vi "LP RT Stream reader State Decide.vi"(8 "error in (no error)":errorcluster, 10 "RefreshRate":i32, 11 "Queue in":refnum<queue>) -> (0 "error out":errorcluster, 1 "Data":variant, 2 "CMD":T1, 3 "queue out":refnum<queue>)   [LabVIEW 2015]
uses:
  Controls/RT Streamer State.ctl
  Controls/RT Streamer Queue element.ctl
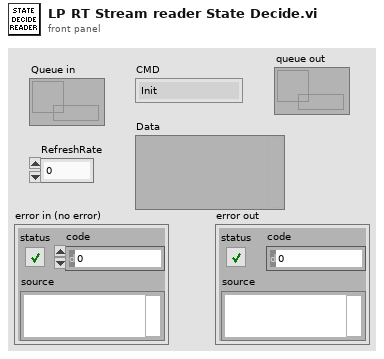
[diagram p1: front panel]
types:
  T1 = typedef "RT Streamer State.ctl" = enum16{"Init", "Idle", "Stream", "Listen", "SetRefrashRate", "SendCmdAck", "SendCmdDone", "SendSysState", "StartRecord", "Error"}
  T2 = typedef "RT Streamer Queue element.ctl" = cluster{"CMD":T1, "Data":variant}
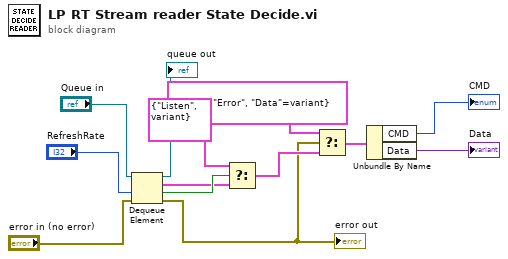
[diagram p0: block diagram]
diagram:
  n1 = Dequeue Element(queue="Queue in", timeout in ms (-1)="RefreshRate", error in (no error)="error in (no error)") -> (queue out=→"queue out":refnum<queue>, element=w6:T2, timed out?=w7:bool, error out=w1:errorcluster)
  "error out" <- w1
  n2 = Select(t=T2 {"CMD"=enum."Listen", "Data"=variant}, s=w7, f=w6) -> (s? t:f=w5:T2)
  n3 = Select(t=T2 {"CMD"=enum."Error", "Data"=variant}, s=w1, f=w5) -> (s? t:f=w9:T2)
  n4 = Unbundle By Name(w9) -> ("CMD"=→"CMD":T1, "Data"=→"Data":variant)
